vi "2017-05-12 Scan+Map - Copy.vi"() -> ()   [LabVIEW 2016]
uses:
  <vilib>/Utility/error.llb/DialogType.ctl
  <vilib>/DAQmx/write.llb/DAQmx Write (Analog DBL 1Chan 1Samp).vi
  <vilib>/DAQmx/create/channels.llb/DAQmx Create Channel (AO-Voltage-Basic).vi
  <vilib>/DAQmx/miscellaneous.llb/DAQmx Fill In Error Info.vi
  <vilib>/Utility/file.llb/Write Delimited Spreadsheet (I64).vi
  HHLib64.dll
panel:
  in  "Path":path
  out "Array 4":dbl[](array[numeric])
  out "Array 3":dbl[][](array[numeric])
  out "Array 2":dbl[](array[numeric])
  out "Array":dbl[][](array[numeric])
  out "Intensity Graph":i32[][](graph)
  out "Count Rates 2":cluster{"rate":i32}
  out "SyncRate 2":i32
  in  "DeviceIndex 2":i32
  in  "Voltage Step":dbl=0.1
  out "Current Voltage":dbl
  out "Next Voltage":dbl
  in  "Wait Time (ms)":dbl=100.0
  in  "Max Voltage 3":dbl=1.0
  in  "Min Voltage Voltage 3":dbl=-1.0
  in  "Scan in X: Set to ao1\nScan in Y: Set to ao0":tag="Dev2/ao0"
  out "Current Voltage 3":dbl
  out "Next Voltage 3":dbl
  in  "Wait Time (ms) 3":dbl=100.0
  in  "Voltage Step 3":dbl=0.1
  in  "Set this opposite to one above":tag="Dev2/ao1"
  in  "Min Voltage Voltage":dbl=-1.0
  in  "Max Voltage":dbl=1.0
  in  "Acq.Time":i32=10000 min=1 max=3600000 step=100
  out "Initialization Status":string
  out "Serial":string
  out "DLL Version":string
  out "DevIdx":dbl
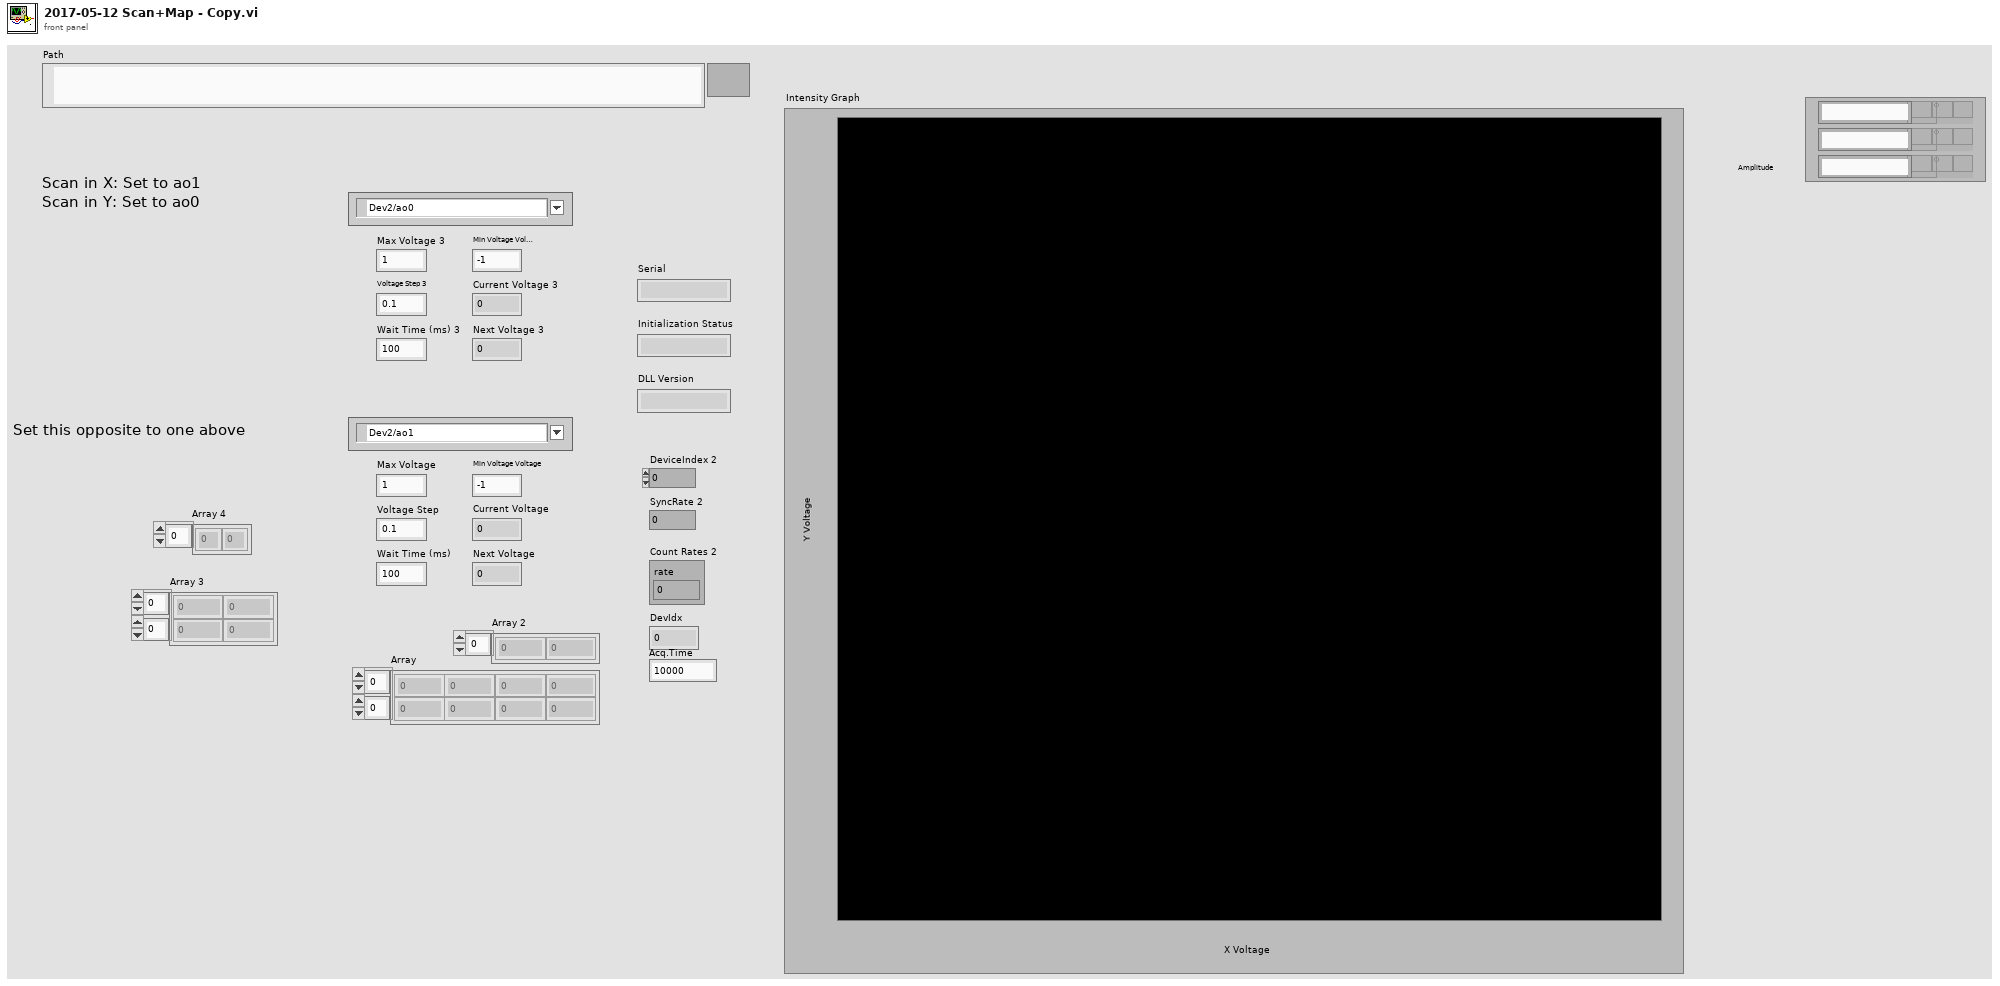
[diagram p1: front panel]
types:
  T1 = typedef "DialogType.ctl" = u16
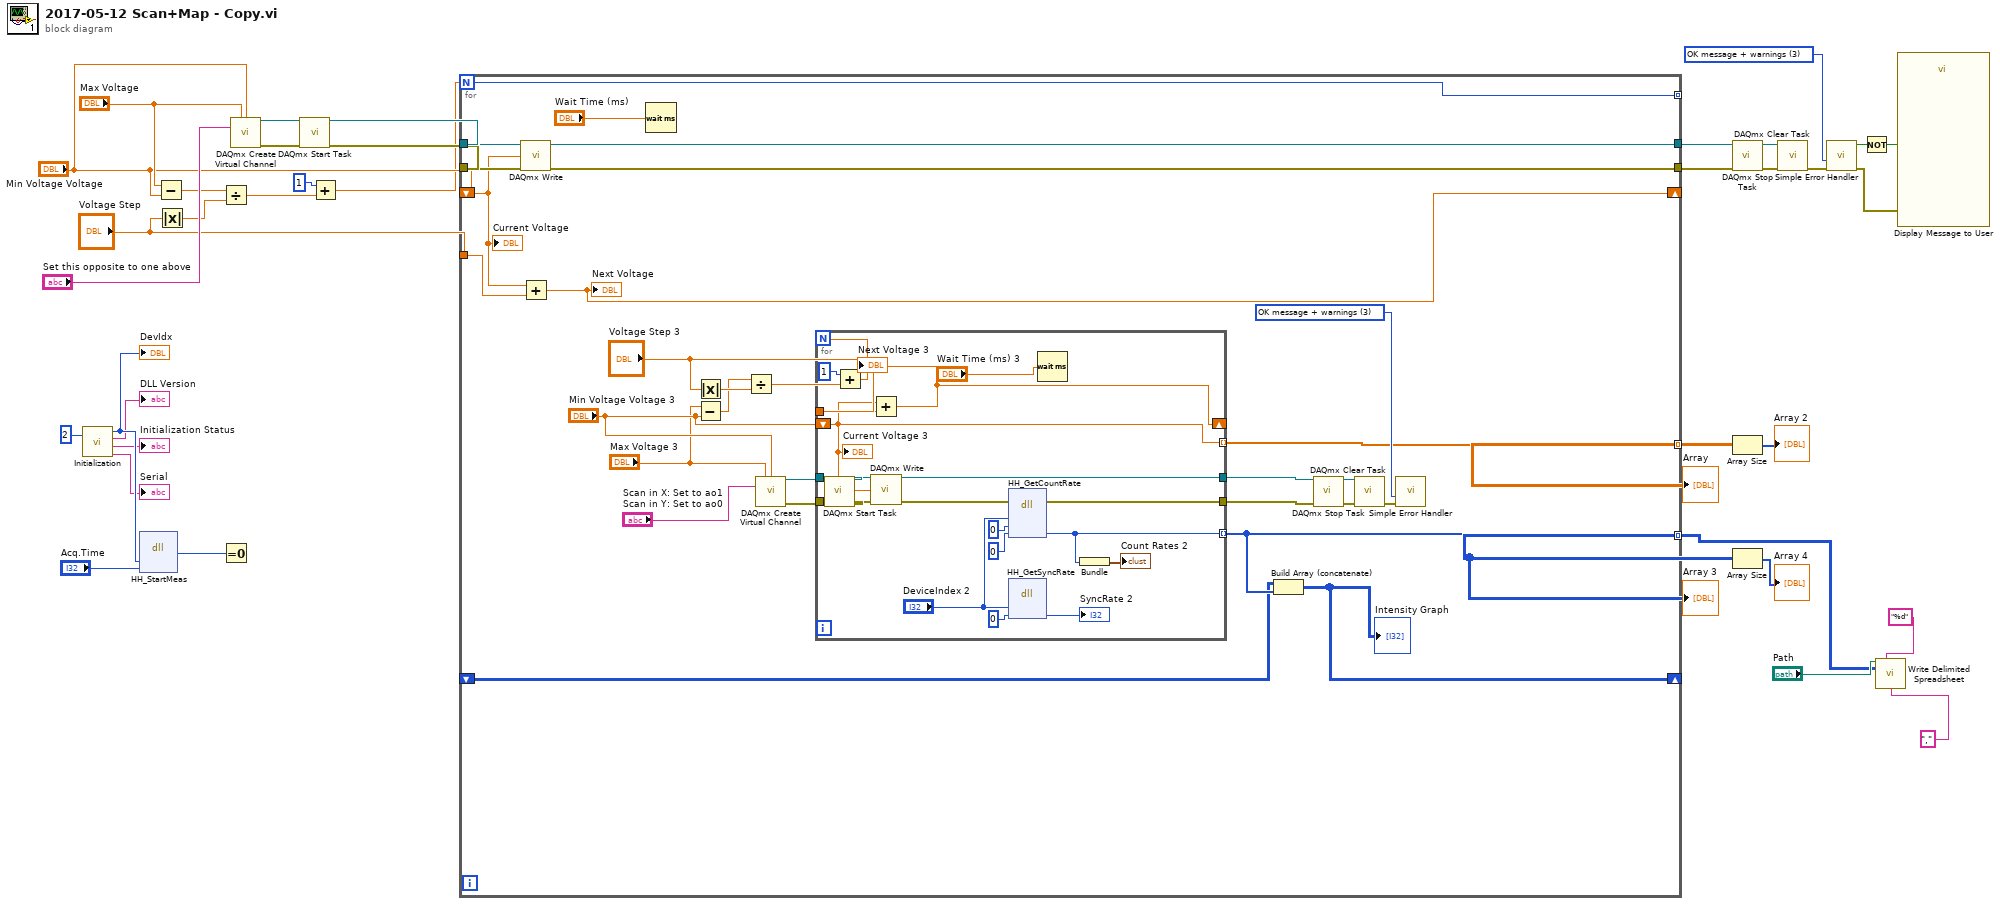
[diagram p0: block diagram]
diagram:
  w27 = T1 3 items=["no dialog", "OK message", "continue or stop message", "OK message + warnings", "continue/stop + warnings"] ("type of dialog (OK msg:1)")
  n1 = call "Initialization.vi"("Mode"=2) -> ("Deviceindex"=w15:i32, "DLL Version"=→"DLL Version":string, "Initialization Status"=→"Initialization Status":string, "Serial[8]"=→"Serial":string)  [unwired: 1 out]
  "DevIdx" <- w15
  n2 = dll-call lib="hhlib64.dll" fn="HH_StartMeas"("devidx"=w15, "tacq"="Acq.Time") -> ("return type"=w14:i32)  [unwired: 5 in, 2 out]
  n3 = Subtract(x="Max Voltage", y="Min Voltage Voltage") -> (x-y=w24:dbl)
  n4 = Absolute Value(x="Voltage Step") -> (abs(x)=w22:dbl)
  n5 = Divide(x=w24, y=w22) -> (x/y=w20:dbl)
  n6 = Equal To 0?(x=w14) -> ()  [unwired: 1 out]
  n7 = call-poly <vilib>:"DAQmx Create Virtual Channel.vi"("maximum value"="Max Voltage", "minimum value"="Min Voltage Voltage", "physical channels"="Set this opposite to one above") -> ("task out"=w35:refnum<k21>, "error out"=w34:errorcluster)  [unwired: 11 in]
  n8 = call <vilib>:"DAQmx Start Task.vi"("task/channels in"=w35, "error in"=w34) -> ("task out"=w33:refnum<k21>, "error out"=w32:errorcluster)  [unwired: 12 in]
  n9 = Add(x=1, y=w20) -> (x+y=w2:dbl)
  n10 = for {
    N: w2 -> [w40]
    tunnel: w33 -> [w68]
    tunnel: w32 -> [w67]
    tunnel: [w66] -> w31
    tunnel: [w64] -> w30
    tunnel: "Voltage Step" -> [w65]
    shift-right: [w63] -> _
    shift-left: "Min Voltage Voltage" -> [w42]
    tunnel: [w41] -> w9 mode=indexing
    tunnel: [w39] -> w1 mode=indexing
    tunnel: [w40] -> _ mode=indexing
    shift-right: [w38] -> _
    shift-left: _ -> [w37]
    w53 = T1 3 items=["no dialog", "OK message", "continue or stop message", "OK message + warnings", "continue/stop + warnings"] ("type of dialog (OK msg:1)")
    n11 = call-poly <vilib>:"DAQmx Write.vi"("task/channels in"=w68, "data"=w42, "error in"=w67) -> ("task out"=w64:refnum<k21>, "error out"=w66:errorcluster)  [unwired: 10 in, 1 out]
    n12 = Add(x=w42, y=w65) -> (x+y=w63:dbl)
    "Next Voltage" <- w63
    n13 = Wait (ms)(milliseconds to wait="Wait Time (ms)") -> ()  [unwired: 1 out]
    n14 = Absolute Value(x="Voltage Step 3") -> (abs(x)=w58:dbl)
    n15 = Subtract(x="Max Voltage 3", y="Min Voltage Voltage 3") -> (x-y=w56:dbl)
    n16 = Divide(x=w56, y=w58) -> (x/y=w60:dbl)
    n17 = call-poly <vilib>:"DAQmx Create Virtual Channel.vi"("maximum value"="Max Voltage 3", "minimum value"="Min Voltage Voltage 3", "physical channels"="Scan in X: Set to ao1\nScan in Y: Set to ao0") -> ("task out"=w45:refnum<k21>, "error out"=w46:errorcluster)  [unwired: 11 in]
    n18 = call <vilib>:"DAQmx Start Task.vi"("task/channels in"=w45, "error in"=w46) -> ("task out"=w47:refnum<k21>, "error out"=w48:errorcluster)  [unwired: 12 in]
    n19 = Add(x=1, y=w60) -> (x+y=w61:dbl)
    n20 = for {
      N: w61 -> [_]
      tunnel: w47 -> [w84]
      tunnel: w48 -> [w83]
      tunnel: [w73] -> w49
      tunnel: [w81] -> w50
      tunnel: "Voltage Step 3" -> [w82]
      shift-right: [w72] -> _
      shift-left: "Min Voltage Voltage 3" -> [w71]
      tunnel: [w71] -> w41 mode=indexing
      tunnel: [w69] -> w39 mode=indexing
      n21 = Add(x=w71, y=w82) -> (x+y=w72:dbl)
      "Next Voltage 3" <- w72
      n22 = call-poly <vilib>:"DAQmx Write.vi"("task/channels in"=w84, "data"=w71, "error in"=w83) -> ("task out"=w81:refnum<k21>, "error out"=w74:errorcluster)  [unwired: 10 in, 1 out]
      n23 = dll-call lib="HHLib64.dll" fn="HH_GetCountRate"(error in=w74, "devidx"="DeviceIndex 2", "channel"=0, "rate"=0) -> (error out=w73:errorcluster, "rate"=w69:i32)  [unwired: 5 in, 1 out]
      n24 = dll-call lib="HHLib64.dll" fn="HH_GetSyncRate"("devidx"="DeviceIndex 2", "rate"=0) -> ("rate"=→"SyncRate 2":i32)  [unwired: 5 in, 2 out]
      n25 = Wait (ms)(milliseconds to wait="Wait Time (ms) 3") -> ()  [unwired: 1 out]
      n26 = Bundle("rate"=w69) -> (→"Count Rates 2":cluster{"rate":i32})  [unwired: 1 in]
      "Current Voltage 3" <- w71
    }
    n27 = Build Array (concatenate)(w37, w39) -> (w38:i32[][])
    "Intensity Graph" <- w38
    n28 = call <vilib>:"DAQmx Stop Task.vi"("task/channels in"=w50, "error in"=w49) -> ("task out"=w52:refnum<k21>, "error out"=w51:errorcluster)  [unwired: 12 in]
    n29 = call <vilib>:"DAQmx Clear Task.vi"("task in"=w52, "error in"=w51) -> ("error out"=w54:errorcluster)  [unwired: 13 in]
    n30 = call <vilib>:"Simple Error Handler.vi"("type of dialog (OK msg:1)"=w53, "error in (no error)"=w54) -> ()  [unwired: 3 in, 5 out]
    "Current Voltage" <- w42
  }
  "Array" <- w9
  "Array 3" <- w1
  n31 = call <vilib>:"DAQmx Stop Task.vi"("task/channels in"=w30, "error in"=w31) -> ("task out"=w28:refnum<k21>, "error out"=w29:errorcluster)  [unwired: 12 in]
  n32 = Array Size(array=w9) -> (size(s)=→"Array 2":i32[])
  n33 = Array Size(array=w1) -> (size(s)=→"Array 4":i32[])
  n34 = call <vilib>:"DAQmx Clear Task.vi"("task in"=w28, "error in"=w29) -> ("error out"=w26:errorcluster)  [unwired: 13 in]
  n35 = call <vilib>:"Simple Error Handler.vi"("type of dialog (OK msg:1)"=w27, "error in (no error)"=w26) -> ("error?"=w18:bool, "error out"=w6:errorcluster)  [unwired: 3 in, 3 out]
  n36 = Not(x=w18) -> (.not. x?=w17:bool)
  n37 = call-poly <vilib>:"Write Delimited Spreadsheet.vi"("file path (dialog if empty)"="Path", "format (%d)"="%d", "2D data"=w1, "delimiter (\\t)"=",") -> ()  [unwired: 10 in, 2 out]
  n38 = call "Display Message to User"("error in (no error)"=w6, "Enable"=w17) -> ()  [unwired: 8 in, 2 out]
